vi "Configure Duration Trigger Source.vi"(0 "VISA resource name":refnum<visa-resource-name>, 5 "Qualifier (0: Greater than)":u16(ring) items=["Greater than", "Less than", "In Range", "Out of Range", "Timeout"], 7 "Duration Pattern Mask (0)":i32, 9 "Duration Pattern Value (0)":i32, 11 "error in (no error)":errorcluster, 12 "Time (1)":dbl=1.0, 13 "Left Range (1)":dbl=1.0, 14 "Right Range (2)":dbl=2.0) -> (4 "VISA resource name out":refnum<visa-resource-name>, 15 "error out":errorcluster)   [LabVIEW 2017, in "Agilent 6000 Series.lvlib"]
doc: "This VI configures the Duration trigger."
uses:
  <instrlib>/Agilent 6000 Series/Agilent 6000 Series.lvlib
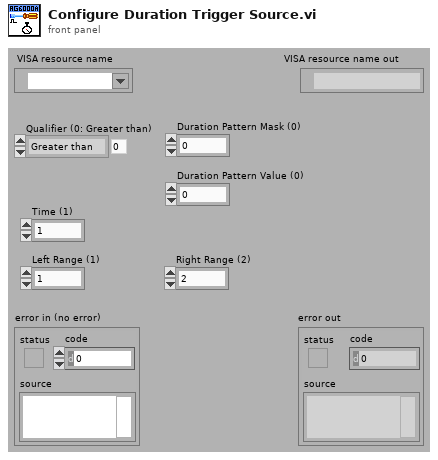
[diagram p1: front panel]
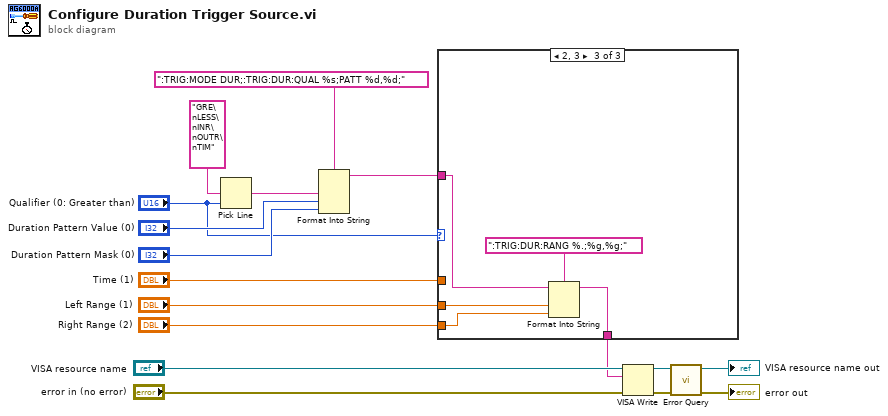
[diagram p0: block diagram]
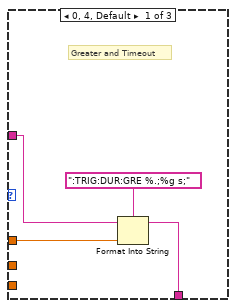
[diagram p2: hidden frame]
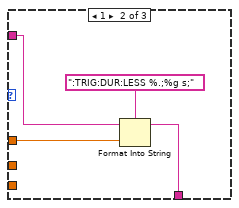
[diagram p3: hidden frame]
diagram:
  n1 = Pick Line(multi-line string="GRE\nLESS\nINR\nOUTR\nTIM", line index="Qualifier (0: Greater than)") -> (output string=w9:string)  [unwired: 1 in]
  n2 = Format Into String(format string=":TRIG:MODE DUR;:TRIG:DUR:QUAL %s;PATT %d,%d;" ("Source Command"), w9, "Duration Pattern Value (0)", "Duration Pattern Mask (0)") -> (resulting string=w4:string)  [unwired: 2 in, 1 out]
  n3 = case shown="2, 3" "Qualifier (0: Greater than)" {
    tunnel: "Time (1)" -> [w20 w24 _]
    tunnel: w4 -> [w19 w23 w29]
    tunnel: "Left Range (1)" -> [_ _ w28]
    tunnel: "Right Range (2)" -> [_ _ w27]
    tunnel: [w18 w22 w26] -> w1
    frame 0, 4, Default {
      # "Greater and Timeout"
      n4 = Format Into String(format string=":TRIG:DUR:GRE %.;%g s;", initial string=w19, w20) -> (resulting string=w18:string)  [unwired: 1 in, 1 out]
    }
    frame 1 {
      n5 = Format Into String(format string=":TRIG:DUR:LESS %.;%g s;", initial string=w23, w24) -> (resulting string=w22:string)  [unwired: 1 in, 1 out]
    }
    frame 2, 3 {
      n6 = Format Into String(format string=":TRIG:DUR:RANG %.;%g,%g;", initial string=w29, w28, w27) -> (resulting string=w26:string)  [unwired: 1 in, 1 out]
    }
  }
  n7 = VISA Write(VISA resource name="VISA resource name", write buffer=w1, error in (no error)="error in (no error)") -> (VISA resource name out=w13:refnum<visa-resource-name>, error out=w12:errorcluster)  [unwired: 1 out]
  n8 = call <instrlib>:"Error Query.vi"("error in (no error)"=w12, "VISA resource name"=w13) -> ("error out"=→"error out":errorcluster, "VISA resource name out"=→"VISA resource name out":refnum<visa-resource-name>)  [unwired: 6 in, 2 out]
